vi "Main.vi"() -> ()   [LabVIEW 2016]
doc: "This Continuous Measurement sample project is based on the Queued Message Handler template.\n\nThe Event Handling Loop generates messages based on user interface actions.\n\nThe Message Handling Loop processes messages generated by the Event Handling Loop, or by other messages. There are also Acquisition and Logging message handling loop subVIs, and a chart updating loop."
uses:
  Acquisition/Hardware Configuration.ctl
  Logging/Logging Configuration.ctl
  controls/UI State.ctl
  <vilib>/Enthought/Python Integration Toolkit/api/Unpack Double.vi
  <vilib>/express/express analysis/Spectral/Block/exnSpectralBlock spectral measurements PSD poly.vi
  <vilib>/express/express analysis/Spectral/Block/exnSpectralBlock spectral measurements PSD DDT.vi
  support/Message Queue/Enqueue Message (Single).vi
  <vilib>/Utility/error.llb/Error Cluster From Error Code.vi
  <vilib>/express/express analysis/Spectral/XNode/ExpressSpectralMeasurementsBlockNode.xnode
  <vilib>/ErrorRing/Error Ring.xnode
  Acquisition/Acquisition.lvlib
  Logging/Logging.lvlib
  Settings/Settings.lvlib
  support/User Event - Stop/User Event - Stop.lvlib
  support/Message Queue/Message Queue.lvlib
  <vilib>/Enthought/Python Integration Toolkit/Python Integration Toolkit.lvlib
panel:
  out "B1S (V)":dbl
  out "X1 2":dynamicdata(graph)=[{"t0"=timestamp(1.8000000000000014 s since 1904-01-01), "dt"=2.0000000000000013, "Y"=array[5000 elements], "attributes"=variant("NI_ChannelName"=variant(string "Dev1/ai0 (Mean)"), "NI_OriginalChannelName"=variant(string "Dev1/ai0"), "NI_UnitDescription"=variant(string "Volts"))}]
  out "X1":dynamicdata(graph)=[{"t0"=timestamp(1.8000000000000014 s since 1904-01-01), "dt"=2.0000000000000013, "Y"=array[5000 elements], "attributes"=variant("NI_ChannelName"=variant(string "Dev1/ai0 (Mean)"), "NI_OriginalChannelName"=variant(string "Dev1/ai0"), "NI_UnitDescription"=variant(string "Volts"))}]
  out "X 4":dynamicdata(graph)
  out "X 3":dynamicdata(graph)
  out "X 2":dynamicdata(graph)
  out "Numeric":dbl
  in  "Step size":dbl
  out "data":i32
  in  "PZTZ+":bool
  in  "PZTZ-":bool
  in  "PZTY+":bool
  in  "PZTX-":bool
  in  "PZTX+":bool
  in  "PZTY-":bool
  out "?":dbl
  out "Input (V)":dbl
  out "Rate (Hz)":dbl
  in  "Stop_Log":bool
  in  "Log":bool
  in  "Exit":bool
  out "Status":string
  in  "Settings":bool
  in  "Stop_Acquire":bool
  in  "Acquire":bool
  out "XY Graph":cluster{"Y":dbl[], "Y":dbl[]}[](graph)
  out "Y":dynamicdata(graph)
  out "X":dynamicdata(graph)
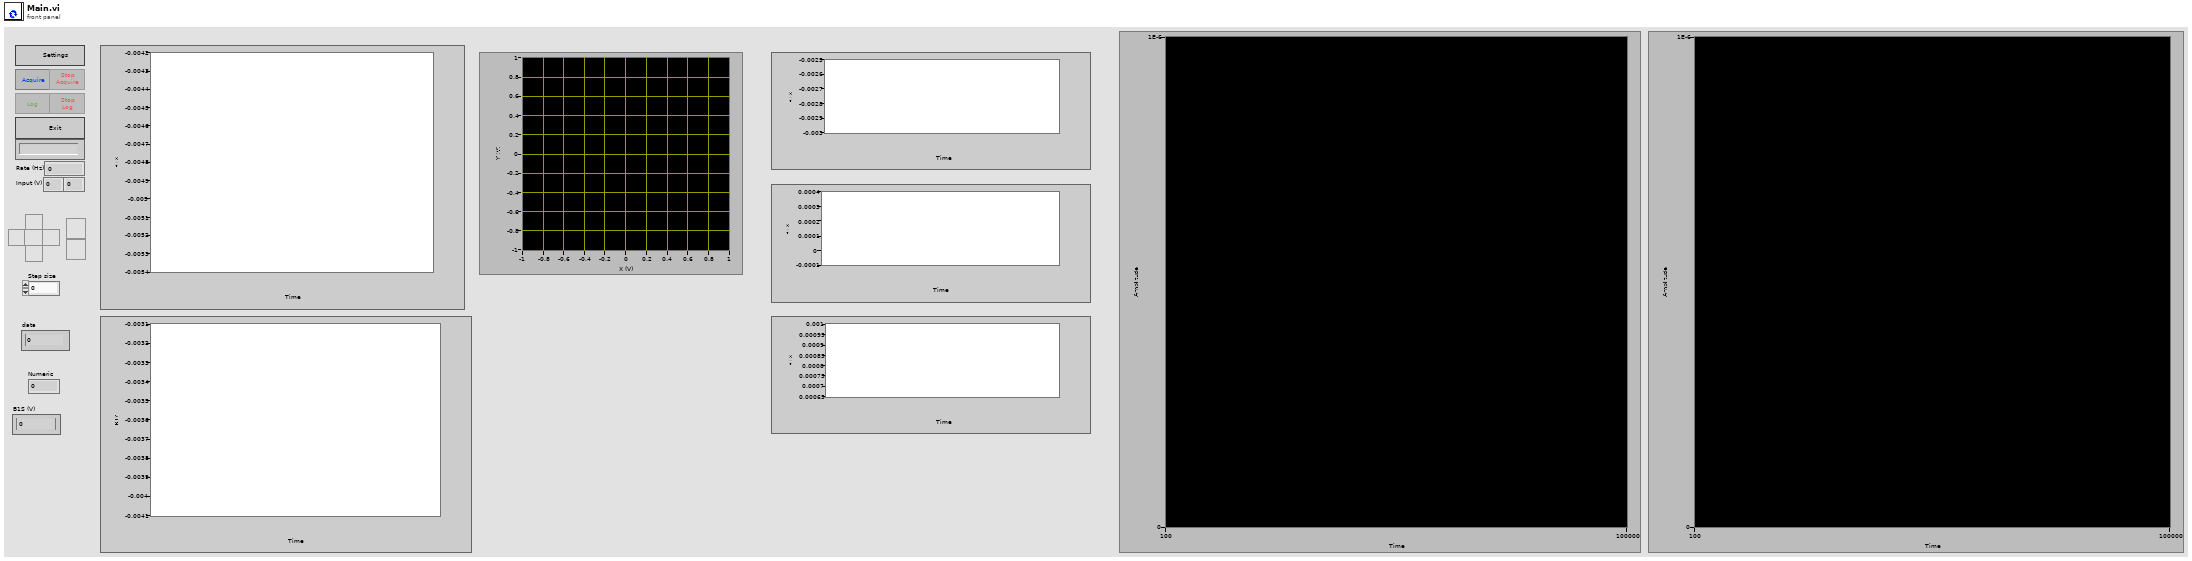
[diagram p1: front panel]
types:
  T1 = typedef "UI State.ctl" = enum16{"Idle", "Acquiring", "Acquiring Stopped", "Logging", "Logging Stopped"}
  T2 = cluster{"Acquire Ref":refnum<vi>, "Log Ref":refnum<vi>, "Stop_Acquire Ref":refnum<vi>, "Settings Ref":refnum<vi>, "Status Ref":refnum<vi>, "Exit Ref":refnum<vi>, "Stop_Log Ref":refnum<vi>}
  T3 = typedef "Acquisition.lvlib/Hardware Configuration.ctl" = cluster{"DAQmx Input":tag, "Max Input":dbl, "Min Input":dbl, "Sample Rate":dbl, "DAQmx Task":refnum<k21>}
  T4 = typedef "Logging.lvlib/Logging Configuration.ctl" = cluster{"Log File Base Path":path, "TDMS File Reference":refnum<k34>, "Channel names":string[], "Author":string, "Description":string}
  T5 = cluster{"Hardware Configuration":T3, "Logging Configuration":T4, "Hardware Configuration 2":cluster{"DAQmx Input":tag, "Max Input":dbl, "Min Input":dbl, "Sample Rate":dbl, "Waveform Type":enum16{"Sine Wave", "Triangle Wave", "Square Wave", "Sawtooth Wave"}, "Sample Rate 2":dbl, "Min Input 2":dbl, "Max Input 2":dbl}}
  T6 = typedef "Message Queue.lvlib/All Message Queues.ctl" = cluster{"UI":refnum<queue>, "Acquisition":refnum<queue>, "Logging":refnum<queue>}
  T7 = typedef "Python Integration Toolkit.lvlib/Session ID.ctl" = u64
  T8 = typedef "Settings.lvlib/Settings.ctl" = cluster{"Hardware Configuration":T3, "Logging Configuration":T4, "PZT Configuration ":T9}
  T9 = typedef "PZT_Control.ctl" = cluster{"DAQmx Output":tag, "PZTX":dbl, "PZTY":dbl, "PZTZ":dbl, "Waveform Type":enum16{"Sine Wave", "Triangle Wave", "Square Wave", "Sawtooth Wave"}, "PZT_Amp":dbl, "PZT_Freq":dbl, "PZT_Phase":dbl}
  T10 = cluster{"Hardware Configuration":T3, "Logging Configuration":cluster{"Log File Base Path":path, "TDMS File Reference":refnum<k34>, "Channel names":string[], "Author":string, "Description":string}, "PZT Configuration ":T9}
  T11 = cluster{"averaging mode":u16, "weighting mode":u16, "number of averages":u32}
  T12 = cluster{"dB On (F)":bool, "unwrap phase (F)":bool, "convert to degree (F)":bool}
  T13 = typedef "Python Integration Toolkit.lvlib/Python Objects.ctl" = variant
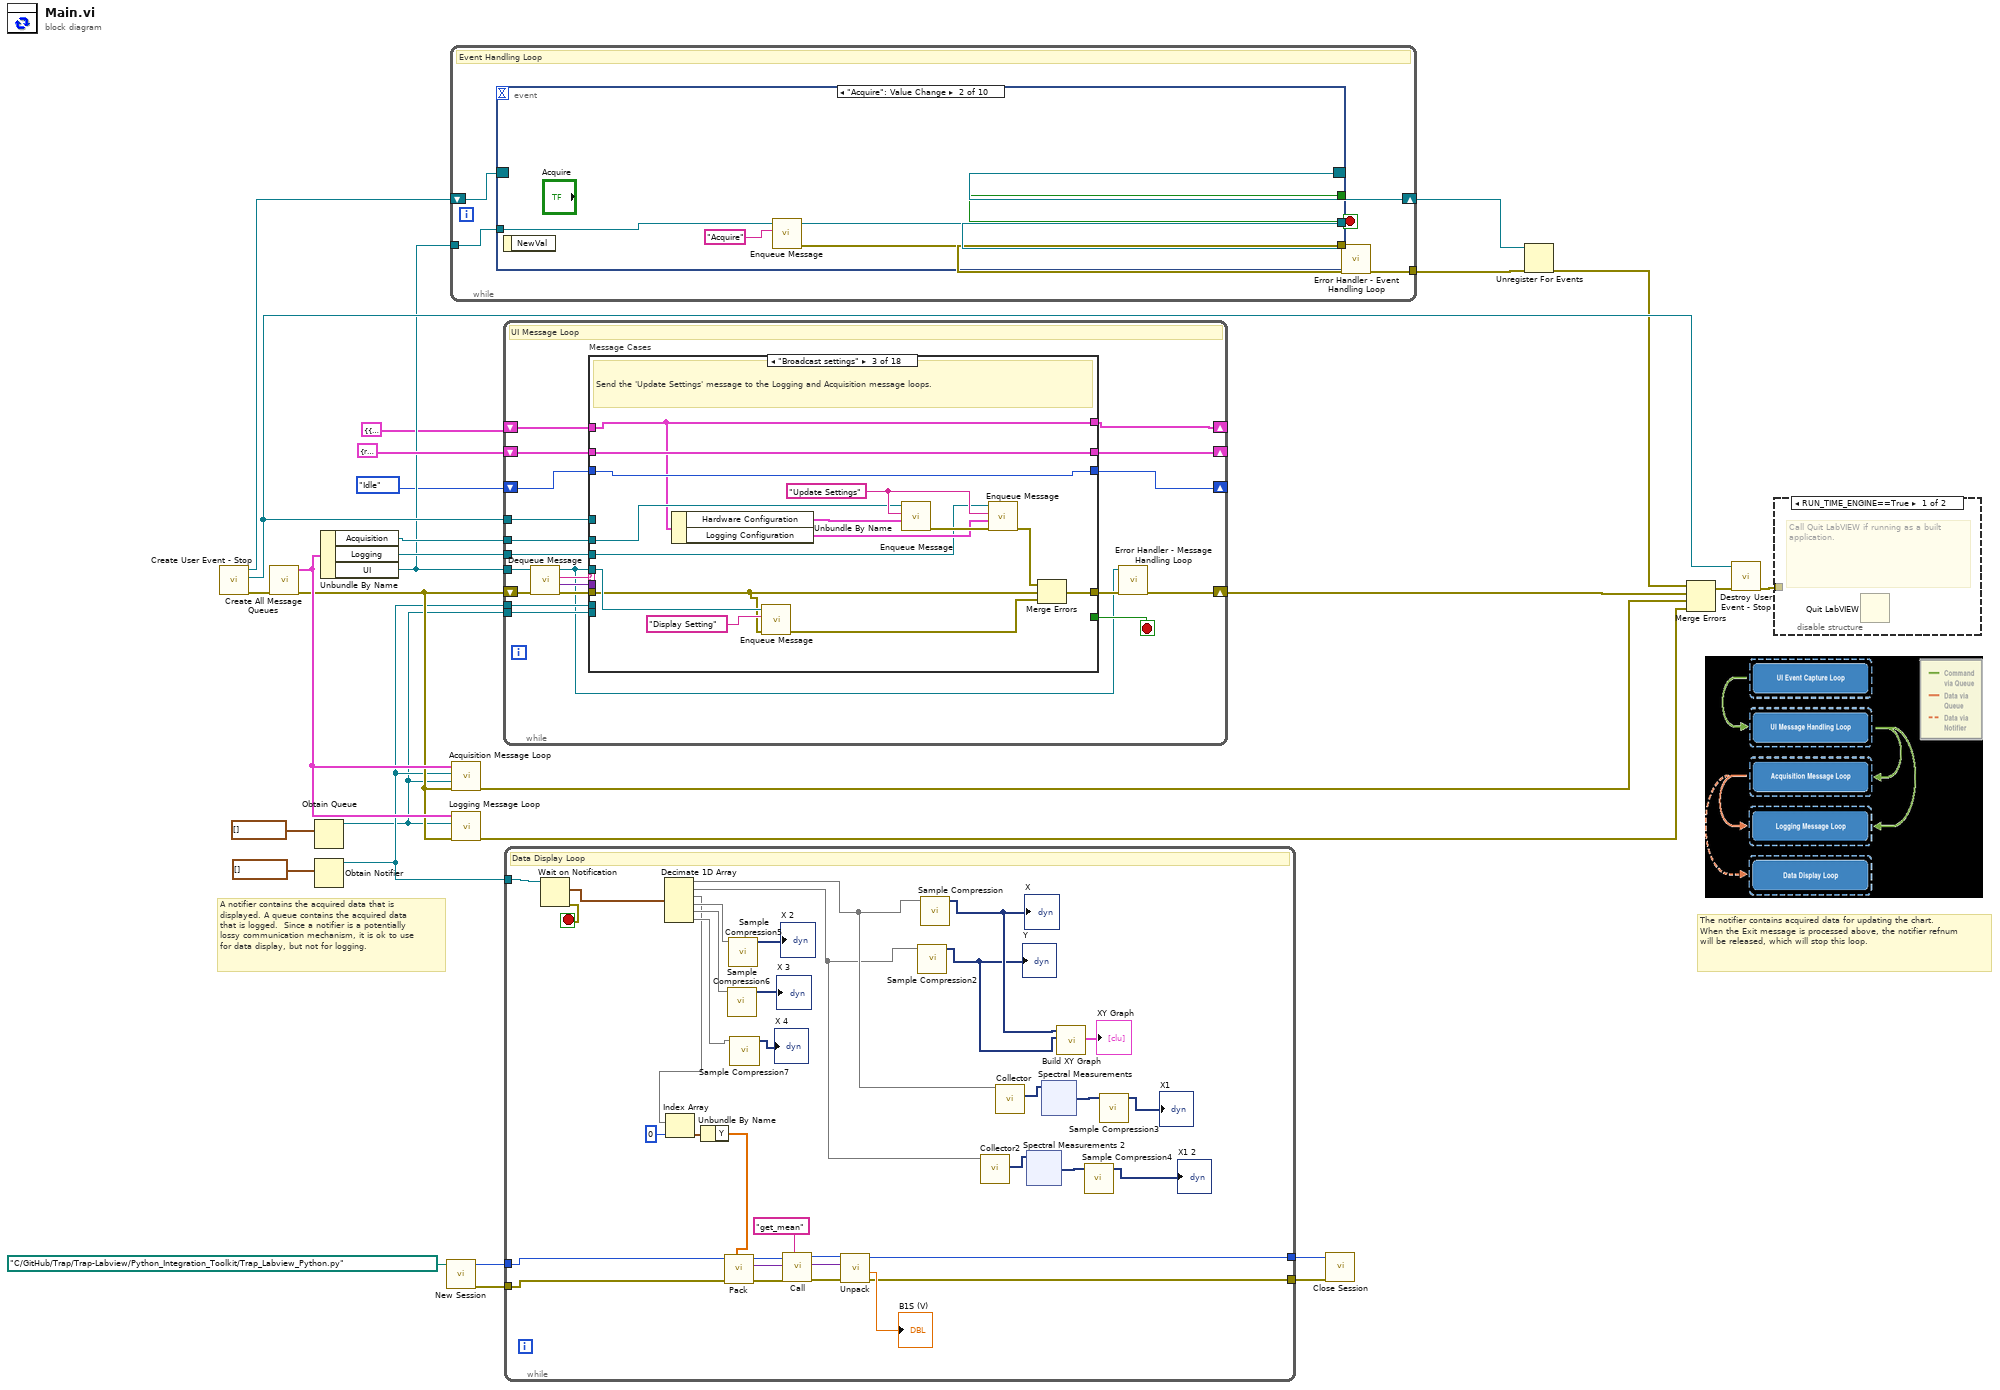
[diagram p0: block diagram]
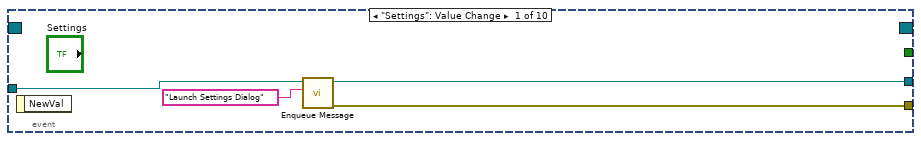
[diagram p3: hidden frame]
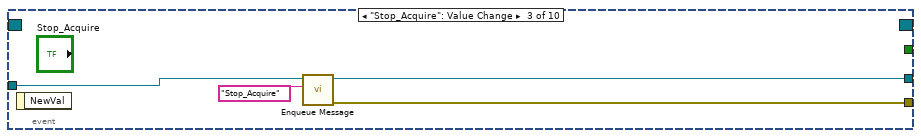
[diagram p4: hidden frame]
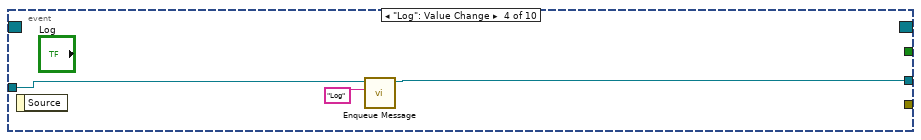
[diagram p5: hidden frame]
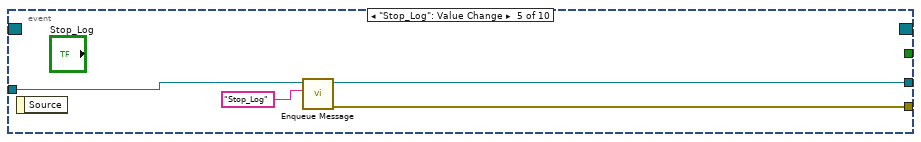
[diagram p6: hidden frame]
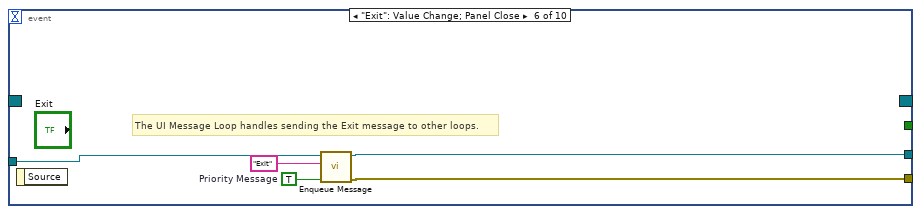
[diagram p7: hidden frame]
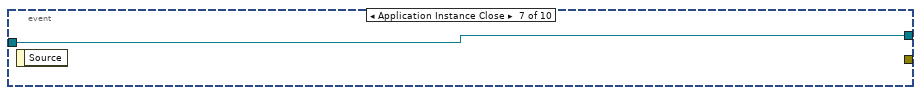
[diagram p8: hidden frame]
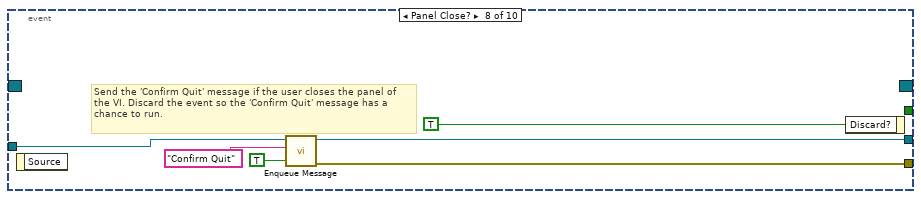
[diagram p9: hidden frame]
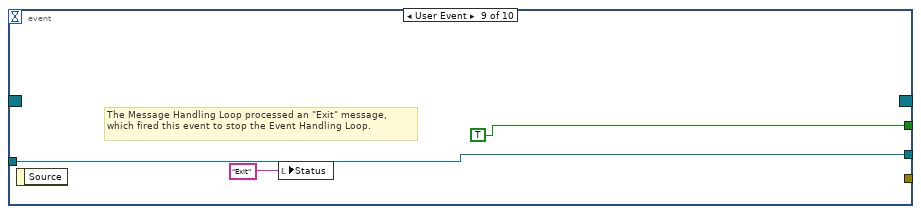
[diagram p10: hidden frame]
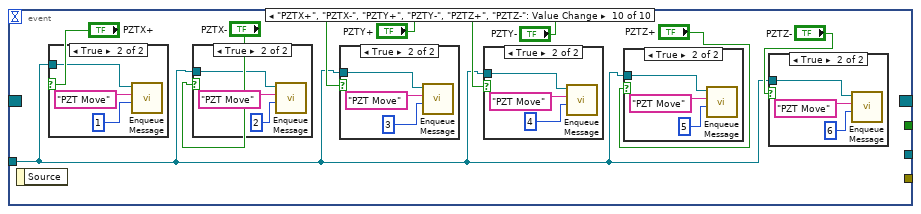
[diagram p11: hidden frame]
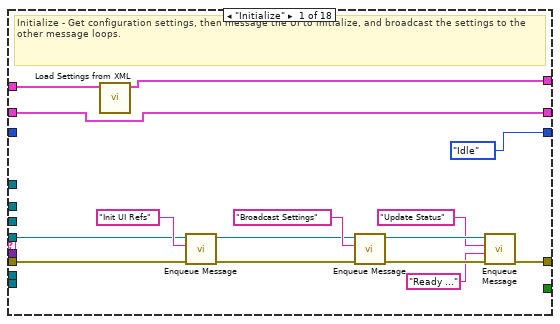
[diagram p18: hidden frame]
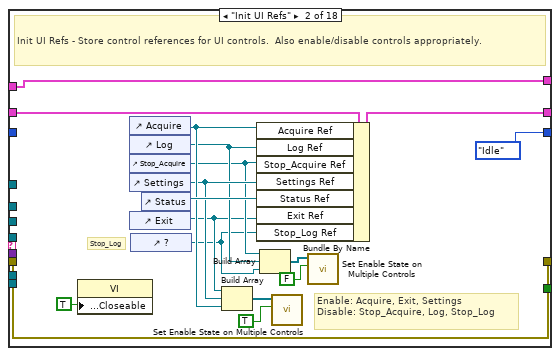
[diagram p19: hidden frame]
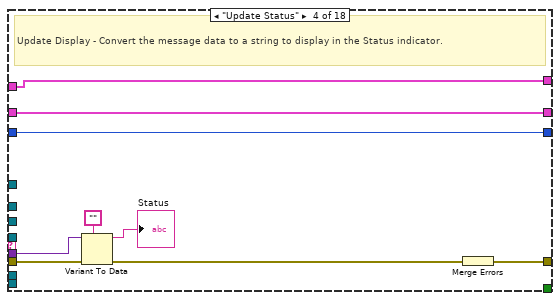
[diagram p20: hidden frame]
diagram:
  # "A notifier contains the acquired data that is displayed. A queue contains the acquired data that is logged.  Since a notifier is a potentially lossy communication mechanism, it is ok to use for data display, but not for logging."
  # "The notifier contains acquired data for updating the chart. When the Exit message is processed above, the notifier refnum will be released, which will stop this loop."
  n1 = call "Create User Event - Stop.vi"() -> ("error out"=w22:errorcluster, "User Event - Stop"=w24:refnum<user-event>, "Stop Event Registration Refnum"=w25:refnum<event-registration>)  [unwired: 9 in]
  n2 = call "Create All Message Queues.vi"("error in (no error)"=w22) -> ("error out"=w19:errorcluster, "Message Queues out"=w21:T6)  [unwired: 9 in]
  n3 = Obtain Queue(element data type=waveform(dbl)[] []) -> (queue out=w6:refnum<queue>)  [unwired: 4 in, 2 out]
  n4 = Obtain Notifier(notification data type=waveform(dbl)[] []) -> (notifier out=w11:refnum<notifier>)  [unwired: 3 in, 2 out]
  n5 = Unbundle By Name(w21) -> ("Acquisition"=w15:refnum<queue>, "Logging"=w14:refnum<queue>, "UI"=w13:refnum<queue>)
  n6 = call <vilib>:"New Session.vi"("Path to Python Module (.py File)"=path "C:/GitHub/Trap/Trap-Labview/Python_Integration_Toolkit/Trap_Labview_Python.py") -> ("error out"=w3:errorcluster, "Session ID out"=w4:T7)  [unwired: 9 in]
  n7 = while {
    tunnel: w13 -> [w34]
    tunnel: [w30] -> w27
    shift-right: [w33] -> w17
    shift-left: w25 -> [w35]
    stop <- w29 stop-if-true
    # "Event Handling Loop"
    n8 = event shown="[1] \"Acquire\": Value Change" {
      selector: w35 -> [_ _ _ _ _ _ _ _ _ _]
      dyn-events: [_ _ _ _ _ _ _ _ _ _] -> w33
      timeout: _ -> [_ _ _ _ _ _ _ _ _ _]
      tunnel: [_ _ _ _ _ _ _ _ TRUE ("Discard?") _] -> w29
      tunnel: w34 -> [w37 w41 w46 w50 w53 w56 w60 w66 w67 w70]
      tunnel: [w39 w43 w45 _ w52 w59 _ w61 _ _] -> w31
      tunnel: [w36 w40 w44 w49 w51 w55 w60 w62 w67 _] -> w32
      event "Settings": Value Change {
        n9 = event-data() -> ()  [unwired: 1 in, 1 out]
        n10 = call-poly "Enqueue Message.vi"("Message"="Launch Settings Dialog", "Message Queue"=w37) -> ("error out"=w39:errorcluster, "dup Message Queue"=w36:refnum<queue>)  [unwired: 8 in]
      }
      event "Acquire": Value Change {
        n11 = event-data() -> ()  [unwired: 1 in, 1 out]
        n12 = call-poly "Enqueue Message.vi"("Message"="Acquire", "Message Queue"=w41) -> ("error out"=w43:errorcluster, "dup Message Queue"=w40:refnum<queue>)  [unwired: 8 in]
      }
      event "Stop_Acquire": Value Change {
        n13 = event-data() -> ()  [unwired: 1 in, 1 out]
        n14 = call-poly "Enqueue Message.vi"("Message"="Stop_Acquire", "Message Queue"=w46) -> ("error out"=w45:errorcluster, "dup Message Queue"=w44:refnum<queue>)  [unwired: 8 in]
      }
      event "Log": Value Change {
        n15 = event-data() -> ()  [unwired: 1 in, 1 out]
        n16 = call-poly "Enqueue Message.vi"("Message"="Log", "Message Queue"=w50) -> ("dup Message Queue"=w49:refnum<queue>)  [unwired: 8 in, 1 out]
      }
      event "Stop_Log": Value Change {
        n17 = event-data() -> ()  [unwired: 1 in, 1 out]
        n18 = call-poly "Enqueue Message.vi"("Message"="Stop_Log", "Message Queue"=w53) -> ("error out"=w52:errorcluster, "dup Message Queue"=w51:refnum<queue>)  [unwired: 8 in]
      }
      event "Exit": Value Change; Panel Close {
        w57 = TRUE  # Priority Message
        # "The UI Message Loop handles sending the Exit message to other loops."
        n19 = event-data() -> ()  [unwired: 1 in, 1 out]
        n20 = call-poly "Enqueue Message.vi"("Priority Message? (F)"=w57, "Message"="Exit", "Message Queue"=w56) -> ("error out"=w59:errorcluster, "dup Message Queue"=w55:refnum<queue>)  [unwired: 7 in]
      }
      event Application Instance Close {
        n21 = event-data() -> ()  [unwired: 1 in, 1 out]
      }
      event Panel Close? {
        # "Send the 'Confirm Quit' message if the user closes the panel of the VI. Discard the event so the 'Confirm Quit' message has a chance to run."
        n22 = event-data() -> ()  [unwired: 1 in, 1 out]
        n23 = call-poly "Enqueue Message.vi"("Priority Message? (F)"=TRUE, "Message"="Confirm Quit", "Message Queue"=w66) -> ("error out"=w61:errorcluster, "dup Message Queue"=w62:refnum<queue>)  [unwired: 7 in]
        n24 = event-data("Discard?"=TRUE) -> ()  [unwired: 1 in, 1 out]
      }
      event User Event {
        # "The Message Handling Loop processed an \"Exit\" message, which fired this event to stop the Event Handling Loop."
        n25 = event-data() -> ()  [unwired: 1 in, 1 out]
        n26 = local write "Status"("Exit" ("Exit String")) -> ()
      }
      event "PZTX+", "PZTX-", "PZTY+", "PZTY-", "PZTZ+", "PZTZ-": Value Change {
        n27 = event-data() -> ()  [unwired: 1 in, 1 out]
        n28 = case shown="True" "PZTX+" {
          tunnel: w70 -> [_ w92]
          frame False {
          }
          frame True {
            n29 = call-poly "Enqueue Message.vi"("Message Data"=1 ("Message"), "Message"="PZT Move", "Message Queue"=w92) -> ()  [unwired: 7 in, 2 out]
          }
        }
        n30 = case shown="True" "PZTX-" {
          tunnel: w70 -> [_ w90]
          frame False {
          }
          frame True {
            n31 = call-poly "Enqueue Message.vi"("Message Data"=2 ("Message"), "Message"="PZT Move", "Message Queue"=w90) -> ()  [unwired: 7 in, 2 out]
          }
        }
        n32 = case shown="True" "PZTY+" {
          tunnel: w70 -> [_ w87]
          frame False {
          }
          frame True {
            n33 = call-poly "Enqueue Message.vi"("Message Data"=3 ("Message"), "Message"="PZT Move", "Message Queue"=w87) -> ()  [unwired: 7 in, 2 out]
          }
        }
        n34 = case shown="True" "PZTY-" {
          tunnel: w70 -> [_ w84]
          frame False {
          }
          frame True {
            n35 = call-poly "Enqueue Message.vi"("Message Data"=4 ("Message"), "Message"="PZT Move", "Message Queue"=w84) -> ()  [unwired: 7 in, 2 out]
          }
        }
        n36 = case shown="True" "PZTZ+" {
          tunnel: w70 -> [_ w81]
          frame False {
          }
          frame True {
            n37 = call-poly "Enqueue Message.vi"("Message Data"=5 ("Message"), "Message"="PZT Move", "Message Queue"=w81) -> ()  [unwired: 7 in, 2 out]
          }
        }
        n38 = case shown="True" "PZTZ-" {
          tunnel: w70 -> [_ w78]
          frame False {
          }
          frame True {
            n39 = call-poly "Enqueue Message.vi"("Message Data"=6 ("Message"), "Message"="PZT Move", "Message Queue"=w78) -> ()  [unwired: 7 in, 2 out]
          }
        }
      }
    }
    n40 = call "Error Handler - Event Handling Loop.vi"("error in (no error)"=w31, "Message Queue"=w32) -> ("dup error in"=w30:errorcluster)  [unwired: 8 in, 1 out]
  }
  n41 = call "Acquisition Message Loop.vi"("error in (no error)"=w19, "Data Queue"=w6, "Data Notifier"=w11, "Message Queues"=w21) -> ("error out"=w23:errorcluster)  [unwired: 7 in]
  n42 = call "Logging Message Loop.vi"("error in (no error)"=w19, "Data Queue"=w6, "Message Queues"=w21) -> ("error out"=w20:errorcluster)  [unwired: 8 in]
  n43 = while {
    tunnel: w13 -> [w108]
    tunnel: w24 -> [w113]
    shift-right: [w99] -> w28
    shift-left: w19 -> [w112]
    shift-right: [w95] -> _
    shift-left: T5 {"Hardware Configuration"={"DAQmx Input"="", "Max Input"=0.0, "Min Input"=0.0, "Sample Rate"=0.0, "DAQmx Task"=""}, "Logging Configuration"={"Log File Base Path"=path "", "TDMS File Reference"=refnum, "Channel names"=[], "Author"="", "Description"=""}, "Hardware Configuration 2"={"DAQmx Input"="", "Max Input"=0.0, "Min Input"=0.0, "Sample Rate"=0.0, "Waveform Type"=enum."Sine Wave", "Sample Rate 2"=0.0, "Min Input 2"=0.0, "Max Input 2"=0.0}} ("Settings") -> [w107]
    shift-right: [w105] -> _
    shift-left: T2 {"Acquire Ref"=refnum, "Log Ref"=refnum, "Stop_Acquire Ref"=refnum, "Settings Ref"=refnum, "Status Ref"=refnum, "Exit Ref"=refnum, "Stop_Log Ref"=refnum} ("Measurement UI Controls") -> [w106]
    tunnel: w15 -> [w104]
    tunnel: w14 -> [w103]
    tunnel: w11 -> [w102]
    tunnel: w6 -> [w101]
    shift-right: [w96] -> _
    shift-left: UI_State."Idle" ("UI State") -> [w97]
    stop <- w114 stop-if-true
    # "UI Message Loop"
    n44 = call "Dequeue Message.vi"("error in (no error)"=w112, "Message Queue"=w108) -> ("error out"=w111:errorcluster, "Message Data"=w109:variant, "Message"=w110:string, "dup Message Queue"=w98:refnum<queue>)  [unwired: 6 in]
    n45 = case "Message Cases" shown="\"Broadcast settings\"" w110 {
      selector: w110 -> [_ _ _ _ _ _ _ _ _ _ _ _ _ _ _ _ _ w394]
      tunnel: w98 -> [w121 _ w151 _ w177 w205 w227 w232 w254 _ w278 w290 w306 w350 _ _ _ _]
      tunnel: w111 -> [w120 w146 w149 w169 w179 w186 w226 w234 w256 w273 w275 w297 w303 w354 w360 w369 w391 _]
      tunnel: [w127 w146 w161 w170 w175 w206 w228 w233 w255 w272 w275 w298 w302 w345 w359 w369 w390 w395] -> w100
      tunnel: [_ _ _ _ _ _ _ _ _ _ _ TRUE _ _ _ _ _ _] -> w114
      tunnel: w109 -> [_ _ _ w168 _ _ _ _ _ _ _ _ _ w353 _ w366 _ _]
      tunnel: w113 -> [_ _ _ _ _ _ _ _ _ _ _ w296 _ _ _ _ _ _]
      tunnel: w107 -> [w116 w130 w147 w162 w172 w185 w207 w229 w237 w257 w274 w281 w300 w343 w356 w363 w384 w392]
      tunnel: w106 -> [w123 w145 w155 w165 w174 w202 w223 w236 w251 w271 w280 w293 w309 w355 w358 w368 w389 w396]
      tunnel: [w123 w144 w155 w165 w174 w202 w223 w236 w251 w271 w280 w293 w309 w355 w358 w368 w389 w396] -> w105
      tunnel: w104 -> [_ _ w154 _ _ w193 w219 _ _ _ _ w292 w305 _ _ _ _ _]
      tunnel: w103 -> [_ _ w153 _ _ _ _ _ w248 w268 _ w291 w304 _ _ _ _ _]
      tunnel: w102 -> [_ _ _ _ _ _ _ _ _ _ _ w289 _ _ _ _ _ _]
      tunnel: w101 -> [_ _ _ _ _ _ _ _ _ _ _ w285 _ _ _ _ _ _]
      tunnel: w97 -> [_ _ w152 w163 w173 _ w208 _ _ _ _ _ w308 w344 w357 w367 w388 w393]
      tunnel: [UI_State."Idle" ("UI State") UI_State."Idle" ("UI State") w152 w163 w173 UI_State."Acquiring" ("UI State") w208 UI_State."Acquiring Stopped" ("UI State") UI_State."Logging" ("UI State") UI_State."Logging Stopped" ("UI State") UI_State."Logging Stopped" ("UI State") UI_State."Idle" ("UI State") w307 w344 w357 w367 w388 w393] -> w96
      tunnel: [w115 w130 w147 w162 w171 w185 w207 w229 w237 w257 w274 w281 w300 w343 w356 w361 w384 w392] -> w95
      frame "Initialize" {
        # "Initialize - Get configuration settings, then message the UI to initialize, and broadcast the settings to the other message loops."
        n46 = call "Load Settings from XML.vi"("Settings in"=w116) -> ("Settings out"=w115:T8)  [unwired: 9 in, 1 out]
        n47 = call-poly "Enqueue Message.vi"("error in (no error)"=w120, "Message"="Init UI Refs", "Message Queue"=w121) -> ("error out"=w118:errorcluster, "dup Message Queue"=w119:refnum<queue>)  [unwired: 7 in]
        n48 = call-poly "Enqueue Message.vi"("error in (no error)"=w118, "Message"="Broadcast Settings", "Message Queue"=w119) -> ("error out"=w129:errorcluster, "dup Message Queue"=w128:refnum<queue>)  [unwired: 7 in]
        n49 = call-poly "Enqueue Message.vi"("error in (no error)"=w129, "Message Data"="Ready ..." ("Ready..."), "Message"="Update Status", "Message Queue"=w128) -> ("error out"=w127:errorcluster)  [unwired: 6 in, 1 out]
      }
      frame "Init UI Refs" {
        # "Stop_Log"
        # "Enable: Acquire, Exit, Settings\nDisable: Stop_Acquire, Log, Stop_Log"
        # "Init UI Refs - Store control references for UI controls.  Also enable/disable controls appropriately."
        n50 = property class="VI"("Front Panel.Closeable"=TRUE ("Front Panel Window:Closeable")) -> ()  [unwired: 2 in, 2 out]
        n51 = control-ref of="Acquire"() -> (w140:refnum<vi>)
        n52 = control-ref of="Log"() -> (w136:refnum<vi>)
        n53 = control-ref of="Stop_Acquire"() -> (w135:refnum<vi>)
        n54 = control-ref of="Settings"() -> (w137:refnum<vi>)
        n55 = control-ref of="Exit"() -> (w132:refnum<vi>)
        n56 = control-ref of="?"() -> (w131:refnum<vi>)
        n57 = control-ref of="Status"() -> (w141:refnum<vi>)
        n58 = Build Array(w132, w137, w140) -> (w139:refnum<vi>[])
        n59 = Bundle By Name(cluster=w145, "Acquire Ref"=w140, "Log Ref"=w136, "Stop_Acquire Ref"=w135, "Settings Ref"=w137, "Status Ref"=w141, "Exit Ref"=w132, "Stop_Log Ref"=w131) -> (w144:T2)
        n60 = Build Array(w135, w136, w131) -> (w134:refnum<vi>[])
        n61 = call "Set Enable State on Multiple Controls.vi"("Enable?"=TRUE, "Controls"=w139) -> ()  [unwired: 10 in]
        n62 = call "Set Enable State on Multiple Controls.vi"("Enable?"=FALSE, "Controls"=w134) -> ()  [unwired: 10 in]
      }
      frame "Broadcast settings" {
        w156 = "Update Settings" ("Message")
        # "Send the 'Update Settings' message to the Logging and Acquisition message loops."
        n63 = Unbundle By Name(w147) -> ("Hardware Configuration"=w159:T3, "Logging Configuration"=w158:T4)
        n64 = call-poly "Enqueue Message.vi"("error in (no error)"=w149, "Message"="Display Setting", "Message Queue"=w151) -> ("error out"=w148:errorcluster)  [unwired: 7 in, 1 out]
        n65 = call-poly "Enqueue Message.vi"("Message Data"=w159, "Message"=w156, "Message Queue"=w154) -> ("error out"=w160:errorcluster)  [unwired: 7 in, 1 out]
        n66 = call-poly "Enqueue Message.vi"("error in (no error)"=w160, "Message Data"=w158, "Message"=w156, "Message Queue"=w153) -> ("error out"=w157:errorcluster)  [unwired: 6 in, 1 out]
        n67 = Merge Errors(w157, w149, w148) -> (w161:errorcluster)
      }
      frame "Update Status" {
        # "Update Display - Convert the message data to a string to display in the Status indicator."
        n68 = Variant To Data(error in=w169, type="", Variant=w168) -> (data=→"Status":string, error out=w166:errorcluster)
        n69 = Merge Errors(w166) -> (w170:errorcluster)
      }
      frame "Launch Settings Dialog" {
        # "Launch the Settings Dialog when the user clicks the 'Settings' button."
        n70 = call "Settings Dialog.vi"("error in (no error)"=w179, "Settings in"=w172) -> ("error out"=w176:errorcluster, "Cancelled?"=w178:bool, "Settings out"=w171:T10)  [unwired: 6 in, 1 out]
        n71 = case shown="False" w178 {
          tunnel: w177 -> [w183 _]
          tunnel: w176 -> [w182 w184]
          tunnel: [w181 w184] -> w175
          frame False {
            n72 = call-poly "Enqueue Message.vi"("error in (no error)"=w182, "Message"="Broadcast Settings", "Message Queue"=w183) -> ("error out"=w181:errorcluster)  [unwired: 7 in, 1 out]
          }
          frame True {
          }
        }
      }
      frame "Acquire" {
        # "Message Acquisition loops to start"
        # "Enable: Stop_Acquire, Log\nDisable: Acquire, Stop_Log, Exit, Settings"
        # "Start - Enable/Disable buttons appropriately for an acquisition that has started, and update status display."
        n73 = Unbundle By Name(w202) -> ("Log Ref"=w190:refnum<vi>, "Stop_Acquire Ref"=w191:refnum<vi>, "Acquire Ref"=w197:refnum<vi>, "Exit Ref"=w196:refnum<vi>, "Settings Ref"=w195:refnum<vi>, "Stop_Log Ref"=w187:refnum<vi>)
        n74 = call-poly "Enqueue Message.vi"("error in (no error)"=w186, "Message Data"="Acquiring data" ("Waiting for trigger"), "Message"="Update Status", "Message Queue"=w205) -> ("error out"=w188:errorcluster)  [unwired: 6 in, 1 out]
        n75 = Build Array(w197, w196, w195, w187) -> (w200:refnum<vi>[])
        n76 = Build Array(w190, w191) -> (w199:refnum<vi>[])
        n77 = call "Set Enable State on Multiple Controls.vi"("Enable?"=TRUE, "Controls"=w199) -> ()  [unwired: 10 in]
        n78 = call "Set Enable State on Multiple Controls.vi"("Enable?"=FALSE, "Controls"=w200) -> ()  [unwired: 10 in]
        n79 = call-poly "Enqueue Message.vi"("error in (no error)"=w188, "Message"="Start", "Message Queue"=w193) -> ("error out"=w194:errorcluster)  [unwired: 7 in, 1 out]
        n80 = Merge Errors(w194) -> (w206:errorcluster)
      }
      frame "Stop_Acquire" {
        # "Message Acquisition loop to stop"
        # "Enable: Acquire, Exit, Settings\nDisable: Stop_Acquire, Log, Stop_Log"
        # "Stop - Enable/Disable buttons appropriately for an acquisition that has stopped, and update status display."
        n81 = Unbundle By Name(w223) -> ("Log Ref"=w217:refnum<vi>, "Stop_Acquire Ref"=w216:refnum<vi>, "Acquire Ref"=w215:refnum<vi>, "Exit Ref"=w214:refnum<vi>, "Settings Ref"=w213:refnum<vi>, "Stop_Log Ref"=w212:refnum<vi>)
        n82 = call-poly "Enqueue Message.vi"("error in (no error)"=w226, "Message Data"="Acquiring Stopped" ("Ready..."), "Message"="Update Status", "Message Queue"=w227) -> ("error out"=w211:errorcluster)  [unwired: 6 in, 1 out]
        n83 = Build Array(w217, w216, w212) -> (w209:refnum<vi>[])
        n84 = Build Array(w215, w214, w213) -> (w210:refnum<vi>[])
        n85 = call "Set Enable State on Multiple Controls.vi"("Enable?"=TRUE, "Controls"=w210) -> ()  [unwired: 10 in]
        n86 = call "Set Enable State on Multiple Controls.vi"("Enable?"=FALSE, "Controls"=w209) -> ()  [unwired: 10 in]
        n87 = call-poly "Enqueue Message.vi"("error in (no error)"=w211, "Message"="Stop", "Message Queue"=w219) -> ("error out"=w220:errorcluster)  [unwired: 7 in, 1 out]
        n88 = Merge Errors(w220) -> (w228:errorcluster)
      }
      frame "Acquisition Stopped" {
        # "Logic for determining what action to take when the acquisition has stopped."
        n89 = call-poly "Enqueue Message.vi"("error in (no error)"=w234, "Message Data"="Ready..." ("Message"), "Message"="Update Status", "Message Queue"=w232) -> ("error out"=w233:errorcluster)  [unwired: 6 in, 1 out]
      }
      frame "Log" {
        # "Enable: Stop_Log\nDisable: Acquire, Stop_Acquire, Exit, Settings, Log"
        # "Duplicate this frame when creating new messages.  Change this comment in the duplicated frame to describe this message."
        n90 = Unbundle By Name(w251) -> ("Stop_Log Ref"=w246:refnum<vi>, "Stop_Acquire Ref"=w244:refnum<vi>, "Acquire Ref"=w243:refnum<vi>, "Exit Ref"=w242:refnum<vi>, "Settings Ref"=w241:refnum<vi>, "Log Ref"=w240:refnum<vi>)
        n91 = call-poly "Enqueue Message.vi"("Message Data"="Logging data" ("Ready..."), "Message"="Update Status", "Message Queue"=w254) -> ()  [unwired: 7 in, 2 out]
        n92 = Build Array(w246) -> (w245:refnum<vi>[])
        n93 = Build Array(w244, w243, w242, w241, w240) -> (w239:refnum<vi>[])
        n94 = call "Set Enable State on Multiple Controls.vi"("Enable?"=TRUE, "Controls"=w245) -> ()  [unwired: 10 in]
        n95 = call "Set Enable State on Multiple Controls.vi"("Enable?"=FALSE, "Controls"=w239) -> ()  [unwired: 10 in]
        n96 = call-poly "Enqueue Message.vi"("Message"="Start", "Message Queue"=w248) -> ()  [unwired: 8 in, 2 out]
        n97 = Merge Errors(w256) -> (w255:errorcluster)
      }
      frame "Stop_Log" {
        # "Message Logging loop to stop"
        # "Enable: Log, Stop_Acquire\nDisable: Acquire, Exit, Settings, Stop_Log"
        # "Duplicate this frame when creating new messages.  Change this comment in the duplicated frame to describe this message."
        n98 = Unbundle By Name(w271) -> ("Stop_Acquire Ref"=w266:refnum<vi>, "Log Ref"=w260:refnum<vi>, "Acquire Ref"=w264:refnum<vi>, "Exit Ref"=w263:refnum<vi>, "Settings Ref"=w262:refnum<vi>, "Stop_Log Ref"=w259:refnum<vi>)
        n99 = Build Array(w266, w260) -> (w265:refnum<vi>[])
        n100 = Build Array(w259, w264, w263, w262) -> (w261:refnum<vi>[])
        n101 = call "Set Enable State on Multiple Controls.vi"("Enable?"=TRUE, "Controls"=w265) -> ()  [unwired: 10 in]
        n102 = call "Set Enable State on Multiple Controls.vi"("Enable?"=FALSE, "Controls"=w261) -> ()  [unwired: 10 in]
        n103 = call-poly "Enqueue Message.vi"("Message"="Stop", "Message Queue"=w268) -> ()  [unwired: 8 in, 2 out]
        n104 = Merge Errors(w273) -> (w272:errorcluster)
      }
      frame "Logging Stopped" {
        # "Logic for determining what action to take when the logging has stopped."
        n105 = call-poly "Enqueue Message.vi"("Message Data"="Acquiring data" ("Ready..."), "Message"="Update Status", "Message Queue"=w278) -> ()  [unwired: 7 in, 2 out]
      }
      frame "Exit" {
        w294 = "Exit" ("Message")
        # "Don't check the error outs. The acquisition and logging queues may have already been released."
        # "Close references owned by the Main VI."
        # "Stop the VI"
        # "Exit - Fire the User Event to stop the Event Handling Loop.  Also send Exit messages to the Acquisition and Logging loops."
        n106 = Release Queue(queue=w290, error in (no error)=w297) -> (error out=w288:errorcluster)  [unwired: 1 in, 2 out]
        n107 = call "Fire User Event - Stop.vi"("User Event - Stop"=w296) -> ("error out"=w295:errorcluster)  [unwired: 10 in]
        n108 = Release Notifier(notifier=w289, error in (no error)=w288) -> (error out=w287:errorcluster)  [unwired: 1 in, 2 out]
        n109 = Release Queue(queue=w285, error in (no error)=w287) -> (error out=w286:errorcluster)  [unwired: 1 in, 2 out]
        n110 = call-poly "Enqueue Message.vi"("Priority Message? (F)"=TRUE, "Message"=w294, "Message Queue"=w292) -> ()  [unwired: 7 in, 2 out]
        n111 = call-poly "Enqueue Message.vi"("Priority Message? (F)"=TRUE, "Message"=w294, "Message Queue"=w291) -> ()  [unwired: 7 in, 2 out]
        n112 = Merge Errors(w295, w286) -> (w298:errorcluster)
      }
      frame "Confirm Quit" {
        # "Confirm Quit - Message that can confirm whether or not the user wants to exit the application."
        n113 = case shown="\"Idle\", Default" w308 {
          tunnel: [w312 w317 w323 w328 w336] -> w301
          tunnel: [UI_State."Idle" ("UI State") UI_State."Acquiring" ("UI State") UI_State."Idle" ("UI State") UI_State."Logging" ("UI State") UI_State."Acquiring" ("UI State")] -> w307
          tunnel: w306 -> [w310 w316 w326 w331 w338]
          tunnel: w305 -> [_ w319 _ _ w341]
          tunnel: w303 -> [_ _ _ _ _]
          tunnel: w304 -> [_ _ _ w334 _]
          frame "Idle", Default {
            # "If 'Confirm Quit' comes in while the system is idle, there is no need for a confirmation message."
            n114 = call-poly "Enqueue Message.vi"("Priority Message? (F)"=TRUE, "Message"="Exit", "Message Queue"=w310) -> ("error out"=w312:errorcluster)  [unwired: 7 in, 1 out]
          }
          frame "Acquiring" {
            n115 = call-poly "Enqueue Message.vi"("Priority Message? (F)"=TRUE, "Message"="Stop", "Message Queue"=w319) -> ("error out"=w318:errorcluster)  [unwired: 7 in, 1 out]
            n116 = call-poly "Enqueue Message.vi"("error in (no error)"=w318, "Message"="Confirm Quit", "Message Queue"=w316) -> ("error out"=w317:errorcluster)  [unwired: 7 in, 1 out]
          }
          frame "Acquiring Stopped" {
            n117 = call-poly "Enqueue Message.vi"("Priority Message? (F)"=TRUE, "Message"="Exit", "Message Queue"=w326) -> ("error out"=w323:errorcluster)  [unwired: 7 in, 1 out]
          }
          frame "Logging" {
            n118 = call-poly "Enqueue Message.vi"("Priority Message? (F)"=TRUE, "Message"="Stop", "Message Queue"=w334) -> ("error out"=w329:errorcluster)  [unwired: 7 in, 1 out]
            n119 = call-poly "Enqueue Message.vi"("error in (no error)"=w329, "Message"="Confirm Quit", "Message Queue"=w331) -> ("error out"=w328:errorcluster)  [unwired: 7 in, 1 out]
          }
          frame "Logging Stopped" {
            n120 = call-poly "Enqueue Message.vi"("Priority Message? (F)"=TRUE, "Message"="Stop", "Message Queue"=w341) -> ()  [unwired: 7 in, 2 out]
            n121 = call-poly "Enqueue Message.vi"("Message"="Confirm Quit", "Message Queue"=w338) -> ("error out"=w336:errorcluster)  [unwired: 8 in, 1 out]
          }
        }
        n122 = Merge Errors(w301, w303) -> (w302:errorcluster)
      }
      frame "Error" {
        # "Error - Check the error message data and respond accordingly. This message is sent by the \"Error Handler\" VIs at the end of each loop in this application."
        n123 = Variant To Data(error in=w354, type=errorcluster {"status"=FALSE, "code"=0, "source"=""} ("error out"), Variant=w353) -> (data=w351:errorcluster, error out=w347:errorcluster)
        n124 = call <vilib>:"Simple Error Handler.vi"("error in (no error)"=w351) -> ()  [unwired: 4 in, 5 out]
        n125 = call-poly "Enqueue Message.vi"("Priority Message? (F)"=TRUE, "Message"="Exit", "Message Queue"=w350) -> ("error out"=w346:errorcluster)  [unwired: 7 in, 1 out]
        n126 = Merge Errors(w346, w347) -> (w345:errorcluster)
      }
      frame "---Copy This Frame---" {
        # "Duplicate this frame when creating new messages.  Change this comment in the duplicated frame to describe this message."
        n127 = Merge Errors(w360) -> (w359:errorcluster)
      }
      frame "PZT Move" {
        n128 = Variant To Data(type=0 ("Message"), Variant=w366) -> (data=w364:i32)  [unwired: 1 in, 1 out]
        "data" <- w364
        n129 = case shown="1" w364 {
          selector: w364 -> [w370 w372 w374 w376 w378 w380 w382]
          tunnel: w363 -> [w371 w373 w375 w377 w379 w381 w383]
          tunnel: [w371 w373 w375 w377 w379 w381 w383] -> w361
          tunnel: "Step size" -> [_ _ _ _ _ _ _]
          frame Default {
            n130 = local write "Numeric"(w370) -> ()
          }
          frame 1 {
            "Numeric" <- w372
          }
          frame 2 {
            n131 = local write "Numeric"(w374) -> ()
          }
          frame 3 {
            n132 = local write "Numeric"(w376) -> ()
          }
          frame 4 {
            n133 = local write "Numeric"(w378) -> ()
          }
          frame 5 {
            n134 = local write "Numeric"(w380) -> ()
          }
          frame 6 {
            n135 = local write "Numeric"(w382) -> ()
          }
        }
      }
      frame "Display Setting" {
        # "Duplicate this frame when creating new messages.  Change this comment in the duplicated frame to describe this message."
        n136 = Unbundle By Name(w384) -> ("Hardware Configuration.Sample Rate"=→"Rate (Hz)":dbl, "Hardware Configuration.Max Input"=→"Input (V)":dbl, "Hardware Configuration.Min Input"=→"?":dbl)
        n137 = Merge Errors(w391) -> (w390:errorcluster)
      }
      frame Default {
        # "'Default' case only runs if there is a message that isn't defined in any of the other cases.  Output a programming error."
        n138 = xnode "Error Ring"("parameter 0"=w394) -> ("error out"=w395:errorcluster)
      }
    }
    n139 = call "Error Handler - Message Handling Loop.vi"("error in (no error)"=w100, "Message Queue"=w98) -> ("dup error in"=w99:errorcluster)  [unwired: 8 in, 1 out]
  }
  n140 = while "Data Display Loop" {
    tunnel: w11 -> [w431]
    tunnel: w4 -> [w420]
    tunnel: w3 -> [w414]
    tunnel: [w405] -> w2
    tunnel: [w404] -> w1
    stop <- w437 stop-if-true
    # "Data Display Loop"
    n141 = Wait on Notification(notifier=w431) -> (notification=w430:waveform(dbl)[], error out=w437:errorcluster)  [unwired: 3 in, 2 out]
    n142 = Decimate 1D Array(w430) -> (w427:waveform(dbl)[], w426:waveform(dbl)[], w407:waveform(dbl)[], w425:waveform(dbl)[], w423:waveform(dbl)[], w410:waveform(dbl)[])
    n143 = Index Array(array=w407, index=0) -> (element=w408:waveform(dbl))
    n144 = Unbundle By Name(w408) -> ("Y"=w406:dbl[])
    n145 = call <vilib>:"Pack.vi"("Argument"=w406, "error in (no error)"=w414, "Session ID"=w420) -> ("error out"=w413:errorcluster, "Python Object References Out"=w418:T13, "Session ID out"=w419:T7)  [unwired: 6 in]
    n146 = call "Sample Compression6"("Signals"=w423) -> ("Mean"=→"X 3":dynamicdata)  [unwired: 8 in, 2 out]
    n147 = call "Sample Compression5"("Signals"=w425) -> ("Mean"=→"X 2":dynamicdata)  [unwired: 8 in, 2 out]
    n148 = call "Sample Compression7"("Signals"=w410) -> ("Mean"=→"X 4":dynamicdata)  [unwired: 8 in, 2 out]
    n149 = call <vilib>:"Call.vi"("Function or Method Name"="get_mean", "error in (no error)"=w413, "Python Object References In"=w418, "Session ID"=w419) -> ("error out"=w412:errorcluster, "Python Object References Out"=w415:T13, "Session ID out"=w416:T7)  [unwired: 5 in]
    n150 = call-poly <vilib>:"Unpack.vi"("error in (no error)"=w412, "Python Object References In"=w415, "Session ID"=w416) -> ("error out"=w404:errorcluster, "Value"=→"B1S (V)":dbl, "Session ID out"=w405:T7)  [unwired: 5 in, 1 out]
    n151 = call "Sample Compression2"("Signals"=w426) -> ("Mean"=w428:dynamicdata)  [unwired: 8 in, 2 out]
    "Y" <- w428
    n152 = call "Sample Compression"("Signals"=w427) -> ("Mean"=w429:dynamicdata)  [unwired: 8 in, 2 out]
    "X" <- w429
    n153 = call "Collector2"("Signals"=w426) -> ("Collected Signals"=w434:dynamicdata)  [unwired: 9 in, 1 out]
    n154 = call "Collector"("Signals"=w427) -> ("Collected Signals"=w439:dynamicdata)  [unwired: 9 in, 1 out]
    n155 = xnode "Spectral Measurements 2"("Signals"=w434) -> ("PSD"=w433:dynamicdata)  [unwired: 1 in, 1 out]
    n156 = xnode "Spectral Measurements"("Signals"=w439) -> ("PSD"=w436:dynamicdata)  [unwired: 1 in, 1 out]
    n157 = call "Build XY Graph"("Y Input"=w428, "X Input"=w429) -> ("XY Graph"=→"XY Graph":cluster{"Y":dbl[], "Y":dbl[]}[])  [unwired: 3 in, 6 out]
    n158 = call "Sample Compression4"("Signals"=w433) -> ("Mean"=→"X1 2":dynamicdata)  [unwired: 8 in, 2 out]
    n159 = call "Sample Compression3"("Signals"=w436) -> ("Mean"=→"X1":dynamicdata)  [unwired: 8 in, 2 out]
  }
  n160 = call <vilib>:"Close Session.vi"("error in (no error)"=w1, "Session ID"=w2) -> ()  [unwired: 9 in, 1 out]
  n161 = Unregister For Events(event registration refnum=w17, error in=w27) -> (error out=w18:errorcluster)
  n162 = Merge Errors(w18, w28, w23, w20) -> (w26:errorcluster)
  n163 = call "Destroy User Event - Stop.vi"("error in (no error)"=w26, "User Event - Stop"=w24) -> ("error out"=w9:errorcluster)  [unwired: 9 in]
  n164 = disable-structure shown="RUN_TIME_ENGINE==True" {
    disable-tunnel: w9 -> [_ _]
    frame condition #0 {
      # "Call Quit LabVIEW if running as a built application."
      n165 = Quit LabVIEW() -> ()  [unwired: 1 in]
    }
    frame condition #1 (active) {
    }
  }
